vi "Vision Research Phantom Series Revision Query.vi"(11 "Error In (no error)":errorcluster) -> (6 "Returned String":string, 8 "Instr Driver Revision":string, 10 "Instr Firmware Revision":string, 15 "Error Out":errorcluster)   [LabVIEW 2013, in "VRI.lvlib"]
doc: "This VI queries the current Vision Research Phantom Series camera firmware revision and instrument driver revision.\n\nThis Instrument Driver's Revision number is 1.0.0\n\nVision Research Phantom Series LabVIEW Driver\nCreated By: BLOOMY CONTROLS, INC\n WINDSOR, CT 06095, USA\n 860-298-9925\n www.bloomy.com\nOriginal Release Date: May, 2004\nOriginally Developed in LabVIEW Version: 7.0\n\nModification History: \n(See the Read Me.txt file for specific changes and additions in each revision)"
uses:
  VRI.lvlib
panel:
  # "For instructions on the use of this VI, press Ctrl+H to display the help window and move the mouse over the icon, controls, and indicators"
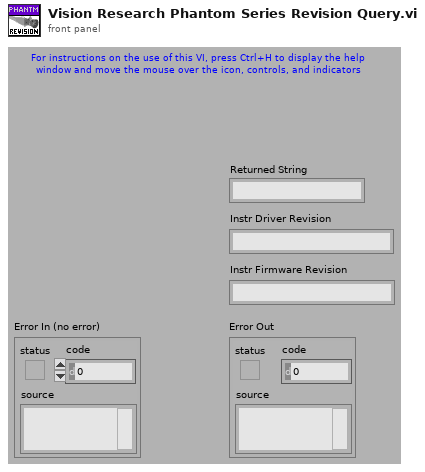
[diagram p1: front panel]
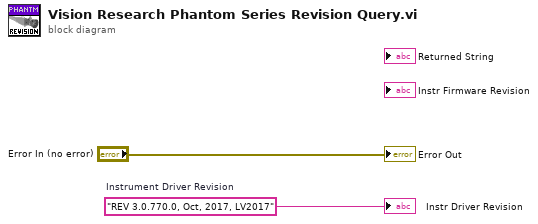
[diagram p0: block diagram]
diagram:
  w2 = "REV 3.0.770.0, Oct, 2017, LV2017"  # Instrument Driver Revision
  "Instr Driver Revision" <- w2
  "Error Out" <- "Error In (no error)"
